vi "STA - Wave V5 Host_Wait_V3.vi"() -> ()   [LabVIEW 2015]
doc: "The continuous acquisition mode tells the FPGA to acquire points indefinitely until a stop command is issued or until an error is encountered (FIFO overflow, module underflow, and so on). \n\nIn this acquisition mode, explicitly call the appropriate rwfm_ConfigTiming VI and set the host application's data buffer to be many times larger than the read size. The examples use a 10X size by default. If the host application's data buffer fills, then the FPGA experiences a FIFO overflow causing the acquisition to stop."
uses:
  <vilib>/LabVIEW Targets/FPGA/cRIO/shared/nicrio_ModuleControls/nicrio_cRIO-9234_ConfigModeRing.ctl
  <vilib>/Platform/TimedLoop/XDataNode/timing_clust.ctl
  <vilib>/Platform/TimedLoop/XDataNode/nitl_modes.ctl
  <vilib>/Platform/TimedLoop/XDataNode/wakeup.ctl
  <vilib>/FPGAPlugInAG/cRIO-9112/niLvFpga_Open_cRIO-9112.vi
  <vilib>/rvi/interface/common/dynamic/niFpgaDynamicAddResources.vi
  <vilib>/Utility/error.llb/Error Cluster From Error Code.vi
  <vilib>/RVI Host/nirviSupport.llb/nirviErrorClusterFromErrorCode.vi
  <vilib>/rvi/errors/niLvFpgaAdjustHostInterfaceError.vi
  <vilib>/FPGAPlugInAG/Dynamic/niLvFpga_Close_Dynamic.vi
  <vilib>/NI/cRIO Wfm/AcqRead(InterleavedSGLs).vi
  <vilib>/rvi/interface/nirviOpenFPGA/nirviOpenFPGA.xnode
  FPGA Bitfiles/STA-WaveformV5_FPGATarget2_[FPGA]DeltaSigMa_sLRIAVfzKK0.lvbitx
  FPGA/[FPGA] DeltaSig Main V5.vi
  <vilib>/rvi/interface/nirviMethod/nirviMethod.xnode
  <vilib>/rvi/interface/nirviCloseFPGA/nirviCloseFPGA.xnode
  <vilib>/Platform/TimedLoop/XDataNode/XDataNode.xnode
  <vilib>/rvi/interface/nirviReadWriteControl/nirviReadWriteControl.xnode
  <vilib>/NI/cRIO Wfm/cRIO Wfm.lvlib
  <vilib>/rvi/interface/nirviMethod/StockFPGA_InlinedMethodWaitForSingleIRQ.vi
  <vilib>/FPGAPlugInAG/Dynamic/niLvFpga_WaitOnIrq_Dynamic.vi
  C:/Program Files (x86)/National Instruments/LabVIEW 2015/ProjectTemplates/Source/cRIOWfm/FPGA/[FPGA] SAR Acq Main.vi
  D/Documents/LabVIEW Data/STA - Waveform V0/FPGA Bitfiles/SARAcqMain_9074.lvbitx
  <vilib>/Platform/TimedLoop/XDataNode/XDNodeRunTimeDep.lvlib
  <vilib>/rvi/interface/Simulation/niFpgaSimulationCallBeginRW.vi
  NiFpgaLv.dll
panel:
  out "Waveform Graph 2":waveform(sgl)[](graph)
  out "error out":errorcluster
  out "Numeric":i32
  in  "stop 2":bool
  out "element out":sgl[](array[numeric])
  in  "Data 5":sgl[][](array[numeric])
  out "Data 3":sgl[](array[numeric])
  in  "Data 2":sgl[](array[numeric])
  in  "Wfm Data":waveform(sgl)[](array[waveform])
  out "Time Measure":dbl
  out "data rate (S/s)":u32
  out "Channel Config":T2(array[cluster]) {"Input Configuration" items=["AC Coupled", "DC Coupled", "IEPE AC Coupled"]}
  in  "Samples per Read":i32=10000
  in  "stop":bool
  out "Waveform Graph":sgl[](graph)
  out "Buffer Backlog":dbl caption="RT Buffer Backlog [%]" format="%#.2g"
  # "Sampling Info"
  # "Channel Info"
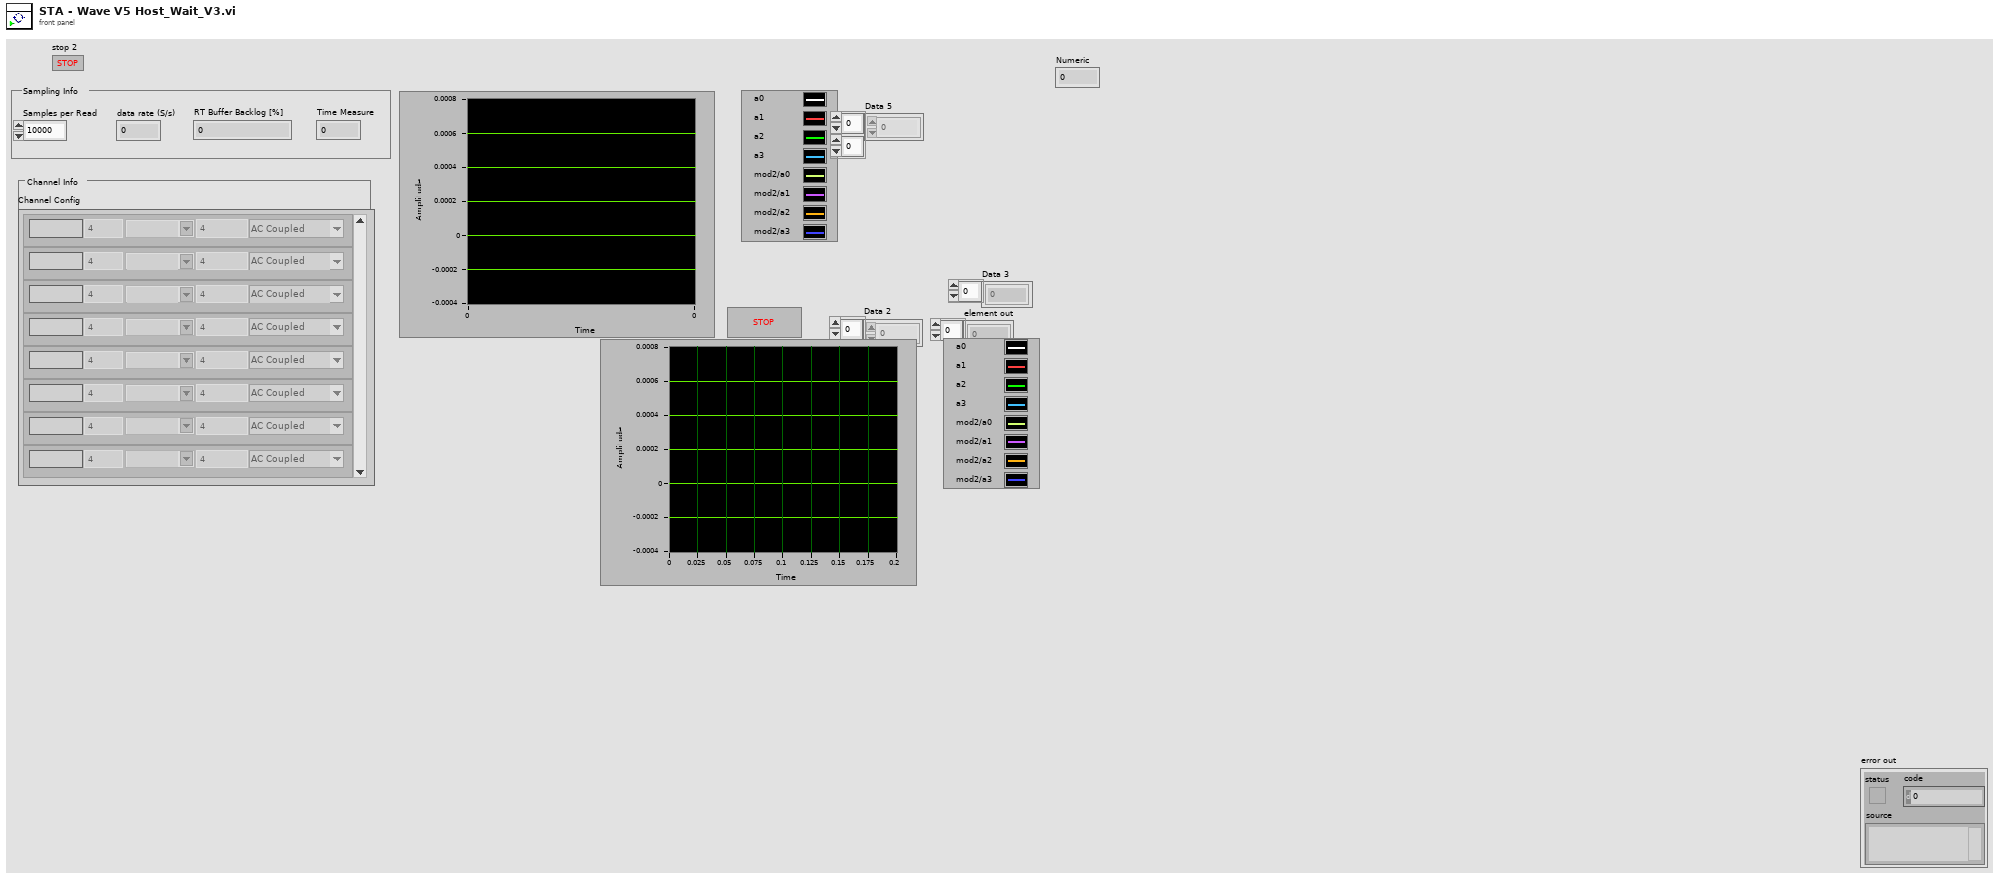
[diagram p1: front panel]
types:
  T1 = typedef "nicrio_cRIO-9234_ConfigModeRing.ctl" = u8
  T2 = cluster{"Channel Name":string, "Sensitivity mV_EU":dbl, "EU":string, "Input Configuration":T1, "dB Ref EU":dbl}[]
  T3 = typedef "XDNodeRunTimeDep.lvlib/timing_clust.ctl" = cluster{"Expected End [f-1]":u64, "Actual End [f-1]":u64, "Finished Late? [f-1]":bool, "Expected End [i-1]":u64, "Actual End [i-1]":u64, "Finished Late? [i-1]":bool, "Expected Start [i]":u64, "Actual Start [i]":u64, "Expected Start [f]":u64, "Actual Start [f]":u64, "Source Name":string, "Structure Name":string, "Period":i64, "Deadline":i64, "Offset":i64, "Start":i64, "Priority":i32, "Timeout":i32, "Mode":T4, "Wakeup Reason":T5, "Error":errorcluster, "Source Type":string, "Secondary Source Type":string, "Global End Time":u64, "Global Start Time":u64, "Frame Duration":u64, "Iteration Duration":u64, "Assigned CPU":i32, "I/O Scan Engine Mode":u32}
  T4 = typedef "XDNodeRunTimeDep.lvlib/nitl_modes.ctl" = enum32{"No Change", "Process missed periods, maintain original phase", "Discard missed periods, maintain original phase", "Process missed periods, ignore original phase", "Discard missed periods, ignore original phase"}
  T5 = typedef "XDNodeRunTimeDep.lvlib/wakeup.ctl" = enum32{"Normal", "Aborted", "Asynchronous wakeup", "Timing source error", "Timed loop error", "Timeout"}
  T6 = typedef "Acquisition and Logging Configuration_Waveform.ctl" = cluster{"Data Rate":T7, "Samples per Read":i32, "Number of Reads to Save":i32, "Data File Name":string, "TDMS Properties":T8[], "Number of Channels":i32, "Trigger - RMS Value":dbl, "Trigger - Channel":i32, "Trigger - Time (Minute)":i32, "Channel Config":cluster{"Channel Name":string, "Sensitivity mV_EU":dbl, "EU":string, "Input Configuration":T1, "dB Ref EU":dbl}[], "data rate (S/s)":u32, "Time Measure":dbl}
  T7 = typedef "nicrio_cRIO-9234_DataRatesRing2.ctl" = u8
  T8 = typedef "TDMS Properties.ctl" = cluster{"Name":string, "Value":string}
  T9 = typedef "cRIO Wfm.lvlib/SamplingInfo.ctl" = cluster{"Number of Channels":i32, "Actual Samp Rate":dbl, "Chan Name Array":string[], "EU Chan Array":string[], "dB Ref Chan Array":dbl[]}
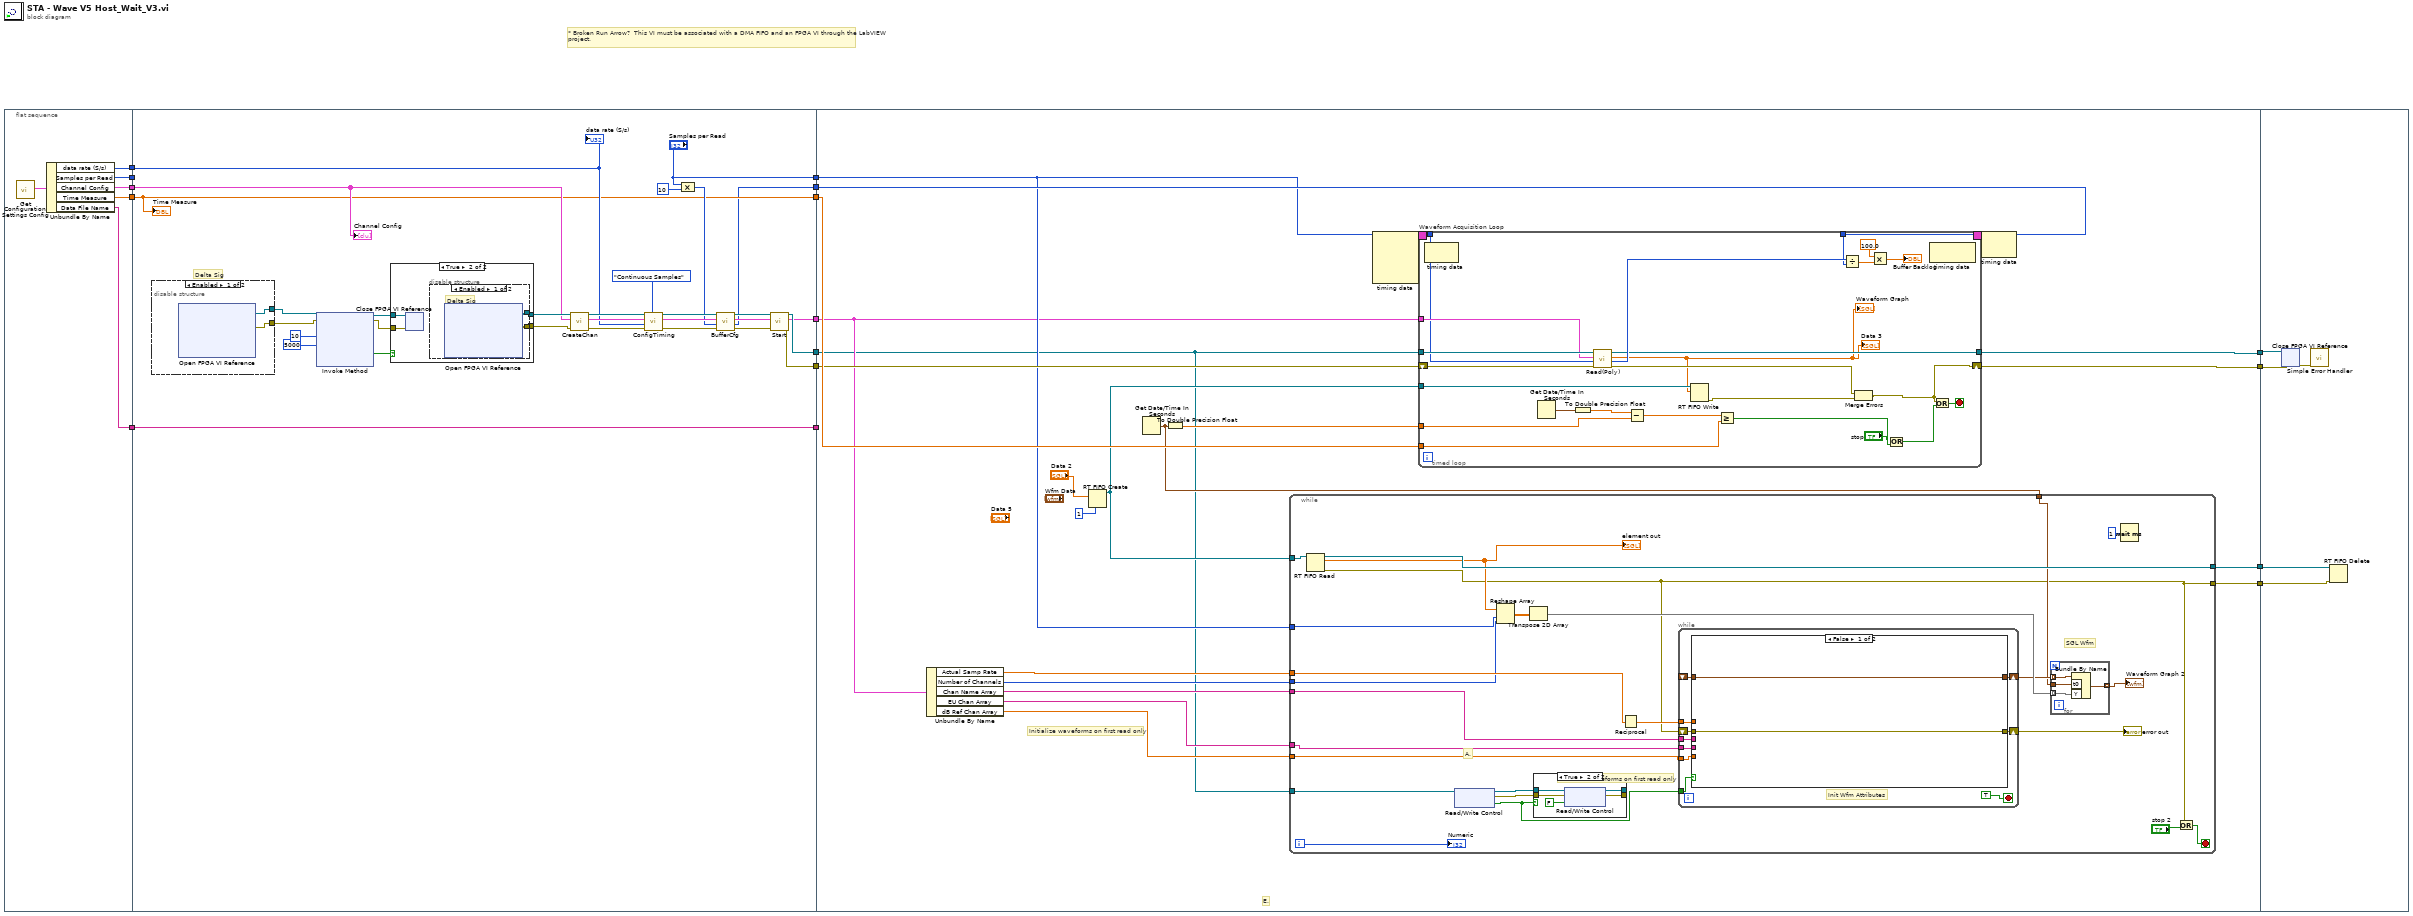
[diagram p0: block diagram]
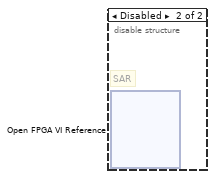
[diagram p2: hidden frame]
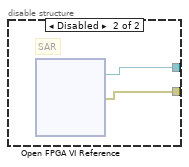
[diagram p4: hidden frame]
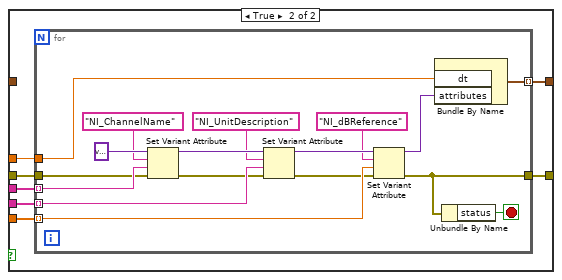
[diagram p6: hidden frame]
diagram:
  # "* Broken Run Arrow?  This VI must be associated with a DMA FIFO and an FPGA VI through the LabVIEW project."
  n1 = flat-sequence {
    tunnel: [w21] -> w16
    tunnel: [w20] -> w15
    tunnel: [w19] -> w14
    tunnel: [w18] -> w13
    tunnel: [w17] -> w4
    tunnel: w16 -> [w33]
    tunnel: w15 -> [_]
    tunnel: w14 -> [w32]
    tunnel: w13 -> [w25]
    tunnel: ["Samples per Read"] -> w12
    tunnel: [w25] -> w11
    tunnel: [w29] -> w10
    tunnel: [w28] -> w9
    tunnel: [w27] -> w8
    tunnel: [w24] -> w7
    tunnel: w4 -> [w23]
    tunnel: [w23] -> w3
    tunnel: w12 -> [w70]
    tunnel: w11 -> [w85]
    tunnel: w10 -> [w67]
    tunnel: w9 -> [w69]
    tunnel: w8 -> [w83]
    tunnel: w7 -> [w84]
    tunnel: [w87] -> w6
    tunnel: [w86] -> w5
    tunnel: w3 -> [_]
    tunnel: [w78] -> w2
    tunnel: [w77] -> w1
    tunnel: w6 -> [w192]
    tunnel: w5 -> [w191]
    tunnel: w2 -> [w190]
    tunnel: w1 -> [w189]
    frame #0 {
      n2 = call "Get Configuration Settings Config.vi"() -> ("Configuration"=w22:T6)  [unwired: 10 in, 1 out]
      n3 = Unbundle By Name(w22) -> ("data rate (S/s)"=w21:u32, "Samples per Read"=w20:i32, "Channel Config"=w19:T2, "Time Measure"=w18:dbl, "Data File Name"=w17:string)
    }
    frame #1 {
      # "Delta Sig"
      n4 = disable-structure shown="Enabled" {
        disable-tunnel: [w54 _] -> w31
        disable-tunnel: [w53 _] -> w30
        frame Enabled {
          n5 = xnode "Open FPGA VI Reference"() -> ("FPGA VI Reference Out"=w54:refnum<k20>, "error out"=w53:errorcluster)  [unwired: 2 in]
        }
        frame Disabled {
          # "SAR"
          n6 = xnode "Open FPGA VI Reference"() -> ("FPGA VI Reference Out"=w56:refnum<k20>, "error out"=w55:errorcluster)  [unwired: 2 in]
        }
      }
      n7 = xnode "Invoke Method"("FPGA VI Reference In"=w31, "error in"=w30, "IRQ Number(s)"=10, "Timeout (ms)"=5000) -> ("FPGA VI Reference Out"=w49:refnum<k20>, "error out"=w50:errorcluster, "Timed Out"=w48:bool)  [unwired: 1 out]
      n8 = case shown="True" w48 {
        tunnel: w49 -> [w58 w62]
        tunnel: w50 -> [w57 w61]
        tunnel: [w58 w60] -> w52
        tunnel: [w57 w59] -> w51
        frame False {
        }
        frame True {
          n9 = xnode "Close FPGA VI Reference"("FPGA VI Reference In"=w62, "error in"=w61) -> ()  [unwired: 1 out]
          n10 = disable-structure shown="Enabled" {
            disable-tunnel: [w64 w66] -> w60
            disable-tunnel: [w63 w65] -> w59
            frame Enabled {
              # "Delta Sig"
              n11 = xnode "Open FPGA VI Reference"() -> ("FPGA VI Reference Out"=w64:refnum<k20>, "error out"=w63:errorcluster)  [unwired: 2 in]
            }
            frame Disabled {
              # "SAR"
              n12 = xnode "Open FPGA VI Reference"() -> ("FPGA VI Reference Out"=w66:refnum<k20>, "error out"=w65:errorcluster)  [unwired: 2 in]
            }
          }
        }
      }
      n13 = call <vilib>:"CreateChan.vi"("Dynamic FPGA Ref"=w52, "Channel Config"=w32, "error in"=w51) -> ("Dynamic FPGA Ref Out"=w39:refnum<k20>, "Sampling Info"=w40:T9, "error out"=w44:errorcluster)  [unwired: 5 in]
      n14 = call <vilib>:"ConfigTiming.vi"("Sample Mode"=enum16{"Finite Samples", "Continuous Samples"}."Continuous Samples", "error in"=w44, "Sample Rate"=w33, "Sampling Info In"=w40, "Dynamic FPGA Ref"=w39) -> ("error out"=w43:errorcluster, "Sampling Info Out"=w42:T9, "Dynamic FPGA Ref Out"=w41:refnum<k20>)  [unwired: 3 in, 1 out]
      n15 = Compound Arithmetic op=MULTIPLY("Samples per Read", 10 ("value")) -> (w37:i32)
      n16 = call <vilib>:"BufferCfg.vi"("error in"=w43, "Buffer Size [Samps per Chan]"=w37, "Sampling Info In"=w42, "Dynamic FPGA Ref"=w41) -> ("error out"=w36:errorcluster, "Buffer Size [Total Samples]"=w24:u32, "Sampling Info Out"=w38:T9, "Dynamic FPGA Ref Out"=w35:refnum<k20>)  [unwired: 4 out]
      n17 = call <vilib>:"Start.vi"("error in"=w36, "Sampling Info In"=w38, "Dynamic FPGA Ref"=w35) -> ("error out"=w27:errorcluster, "Sampling Info Out"=w28:T9, "Dynamic FPGA Ref Out"=w29:refnum<k20>)  [unwired: 6 out]
      "Channel Config" <- w32
      "data rate (S/s)" <- w33
      "Time Measure" <- w25
    }
    frame #2 {
      # "Initialize waveforms on first read only"
      # "E."
      n18 = Unbundle By Name(w69) -> ("Actual Samp Rate"=w73:dbl, "Number of Channels"=w71:i32, "Chan Name Array"=w72:string[], "EU Chan Array"=w74:string[], "dB Ref Chan Array"=w75:dbl[])
      n19 = RT FIFO Create(1:"Data 2", 5:u32 1 ("datapoints in waveform (1)")) -> (8:w79:refnum<k33>)  [unwired: 6 in, 2 out]
      n20 = Get Date/Time In Seconds() -> (seconds since 1Jan1904=w68:timestamp)
      n21 = To Double Precision Float(number=w68) -> (double precision float=w88:dbl)
      n22 = while {
        tunnel: w79 -> [w113]
        tunnel: [w112] -> w78
        tunnel: [w94] -> w77
        tunnel: w75 -> [w103]
        tunnel: w74 -> [w104]
        tunnel: w73 -> [w102]
        tunnel: w72 -> [w100]
        tunnel: w71 -> [w99]
        tunnel: w70 -> [w98]
        tunnel: w68 -> [w95]
        tunnel: w67 -> [w90]
        i -> [w109]
        stop <- w110 stop-if-true
        # "A."
        # "Initialize waveforms on first read only"
        # "SGL Wfm"
        n23 = RT FIFO Read(0:w113) -> (8:w112:refnum<k33>, 9:w105:sgl[], 11:w94:errorcluster)  [unwired: 3 in, 2 out]
        "element out" <- w105
        n24 = xnode "Read/Write Control"("FPGA VI Reference In"=w90) -> ("FPGA VI Reference Out"=w92:refnum<k20>, "error out"=w93:errorcluster, "First Read"=w91:bool)  [unwired: 1 in]
        n25 = Reshape Array(w105, w98, w99) -> (w107:sgl[][])
        n26 = Transpose 2D Array(2D array=w107) -> (transposed array=w106:sgl[][])
        n27 = case shown="True" w91 {
          tunnel: w92 -> [w115 w120]
          tunnel: [w115 w119] -> _
          tunnel: w93 -> [w114 w118]
          tunnel: [w114 w117] -> _
          frame False {
          }
          frame True {
            n28 = xnode "Read/Write Control"("FPGA VI Reference In"=w120, "error in"=w118, "First Read"=FALSE) -> ("FPGA VI Reference Out"=w119:refnum<k20>, "error out"=w117:errorcluster)
          }
        }
        n29 = Reciprocal(x=w102) -> (1/x=w101:dbl)
        n30 = while {
          tunnel: w104 -> [w130]
          tunnel: w103 -> [w129]
          tunnel: w101 -> [w128]
          tunnel: w100 -> [w127]
          shift-right: [w121] -> w96
          shift-left: w94 -> [w125]
          shift-right: [w126] -> w97
          shift-left: _ -> [w123]
          tunnel: w91 -> [w122]
          stop <- TRUE stop-if-true
          # "Init Wfm Attributes"
          n31 = case shown="False" w122 {
            tunnel: w128 -> [_ w139]
            tunnel: w129 -> [_ w138]
            tunnel: w130 -> [_ w136]
            tunnel: w127 -> [_ w135]
            tunnel: [w132 w134] -> w126
            tunnel: w125 -> [w131 w133]
            tunnel: w123 -> [w132 _]
            tunnel: [w131 w137] -> w121
            frame False {
            }
            frame True {
              n32 = for {
                tunnel: w139 -> [w156]
                tunnel: [w155] -> w134 mode=indexing
                tunnel: w136 -> [w153] mode=indexing
                tunnel: w138 -> [w150] mode=indexing
                tunnel: [w152] -> w137
                tunnel: w135 -> [w141] mode=indexing
                tunnel: w133 -> [w140]
                stop <- w151 stop-if-true
                n33 = Set Variant Attribute(Variant=variant ("variant out"), name="NI_ChannelName", value=w141, error in=w140) -> (Variant out=w146:variant, error out=w148:errorcluster)  [unwired: 1 out]
                n34 = Set Variant Attribute(Variant=w146, name="NI_UnitDescription", value=w153, error in=w148) -> (Variant out=w147:variant, error out=w149:errorcluster)  [unwired: 1 out]
                n35 = Set Variant Attribute(Variant=w147, name="NI_dBReference", value=w150, error in=w149) -> (Variant out=w154:variant, error out=w152:errorcluster)  [unwired: 1 out]
                n36 = Bundle By Name("dt"=w156, "attributes"=w154) -> (w155:waveform(sgl))  [unwired: 1 out]
                n37 = Unbundle By Name(w152) -> ("status"=w151:bool)
              }
            }
          }
        }
        "error out" <- w96
        n38 = for {
          tunnel: w97 -> [w160] mode=indexing
          tunnel: w95 -> [w159]
          tunnel: [w158] -> w89 mode=indexing
          tunnel: w106 -> [w157] mode=indexing
          n39 = Bundle By Name(cluster=w160, "t0"=w159, "Y"=w157) -> (w158:waveform(sgl))
        }
        "Waveform Graph 2" <- w89
        n40 = Wait (ms)(milliseconds to wait=u32 1) -> ()  [unwired: 1 out]
        n41 = Or(x=w94, y="stop 2") -> (x .or. y?=w110:bool)
        "Numeric" <- w109
      }
      n42 = node-c288() -> (w81:T3)  [unwired: 4 in]
      n43 = timed-loop "Waveform Acquisition Loop" {
        tunnel: [w178] -> w87
        shift-right: [w176] -> w86
        shift-left: w83 -> [w184]
        tunnel: w88 -> [w169]
        tunnel: w85 -> [w168]
        tunnel: w67 -> [w167]
        tunnel: w69 -> [w166]
        tunnel: w70 -> [w165]
        tunnel: w84 -> [w164]
        tunnel: w79 -> [w163]
        timing: w81 -> [_]
        timing-out: [_] -> w80
        stop <- w179 stop-if-true
        n44 = node-c288() -> ()  [unwired: 1 in, 1 out]
        n45 = Get Date/Time In Seconds() -> (seconds since 1Jan1904=w171:timestamp)
        n46 = To Double Precision Float(number=w171) -> (double precision float=w170:dbl)
        n47 = call-poly <vilib>:"Read(Poly).vi"("error in"=w184, "Samps Read per Chan"=w165, "Sampling Info"=w166, "Dynamic FPGA Ref"=w167) -> ("error out"=w177:errorcluster, "Samples Remaining"=w183:u32, "Data"=w161:sgl[], "Dynamic FPGA Ref Out"=w178:refnum<k20>)  [unwired: 4 in]
        "Waveform Graph" <- w161
        "Data 3" <- w161
        n48 = Subtract(x=w170, y=w169) -> (x-y=w172:dbl)
        n49 = RT FIFO Write(0:w163, 1:w161) -> (11:w162:errorcluster)  [unwired: 3 in, 3 out]
        n50 = Greater Or Equal?(x=w172, y=w168) -> (x >= y?=w175:bool)
        n51 = Divide(x=w183, y=w164) -> (x/y=w182:dbl)
        n52 = Merge Errors(w177, w162) -> (w176:errorcluster)
        n53 = Multiply(x=100.0, y=w182) -> (x*y=→"Buffer Backlog":dbl)
        n54 = Or(x="stop", y=w175) -> (x .or. y?=w173:bool)
        n55 = node-c288() -> ()  [unwired: 1 in, 1 out]
        n56 = Or(x=w176, y=w173) -> (x .or. y?=w179:bool)
      }
      n57 = node-c288(w80) -> ()  [unwired: 1 out]
    }
    frame #3 {
      n58 = xnode "Close FPGA VI Reference"("FPGA VI Reference In"=w192, "error in"=w191) -> ("error out"=w193:errorcluster)
      n59 = call <vilib>:"Simple Error Handler.vi"("error in (no error)"=w193) -> ()  [unwired: 1 in, 8 out]
      n60 = RT FIFO Delete(0:w190, 3:w189) -> ()  [unwired: 1 in, 1 out]
    }
  }
